vi "fake SampleRotator module.vi"(10 "Top":refnum<queue>, 11 "Rotator":refnum<queue>) -> (2 "deviceHandle":i32, 3 "Initialized":bool)   [LabVIEW 2022 SP3, in "SampleRotator.lvlib"]
doc: "This is a main VI of module for Sample rotator. It recives and executes commands, which comes from master controller. \nCommands and responses:\n\n/* */\nInitialize(path to driver DLL); -> Initialized(Contoller info<devN, devT, ID, Serial, Addr, connected?>);\n\n/* */\nUpdate(); -> Update(axis status<axis info, position, frequency, voltage>);\n\n/* */\nSetParameters(parameters<freq[Hz]; ampl[V]; offset[V]; tolerance[um]>); -> ParametersSet(parameters<freq; amp; offset; tolerance>);\n\n/* */\nSetPositon(positionToSet<relative?, double>) -> PositionSet(position to set<relative?, doubele);\n\n/* */\nEnd(), -> Disconnected();"
uses:
  SampleRotator.lvlib
  ctl/Rotator controller info.ctl
  ctl/Axis status.ctl
  Messenger service/Data types/Module name.ctl
  ctl/Motion Properties.ctl
  ctl/Positoin to set.ctl
  ctl/Rotator commands.ctl
panel:
  in  "Axis status in":T1={"Axis status"={"Connected"=TRUE, "Enabled"=FALSE, "Moving"=FALSE, "Target"=FALSE, "EndForward"=FALSE, "EndBackarwd"=FALSE, "Error"=FALSE}, "Position [°]"=0.0, "Frequency [Hz]"=1000.0, "Voltage [V]"=10.0, "Capacitance[uF]"=0.0, "Name"="", "ActuatorType"=0, "DC offset [V]"=0.0, "Tolerance [m°]"=0.0, "Index"=0} {"Index" items=["1", "2", "3"]; "ActuatorType" items=["Linear", "Rotator", "Goniometer"]}
  in  "controller info in":T2={"deviceNumber"=0, "DeviceType"=0, "ID"=0, "Serial"="", "Address"="FAKE", "connected"=TRUE} {"DeviceType" items=["ANC350res", "ANC350num", "ANC350fps", "No device / invalid"]; "ID" format="%x"}
  out "capacity":dbl
  out "wrong capacity":bool
  out "Axis status":T1 {"Index" items=["1", "2", "3"]; "ActuatorType" items=["Linear", "Rotator", "Goniometer"]}
  out "path to dll":path
  out "controller info":T2 {"DeviceType" items=["ANC350res", "ANC350num", "ANC350fps", "No device / invalid"]; "ID" format="%x"}
  out "ANC350v4 found":u32
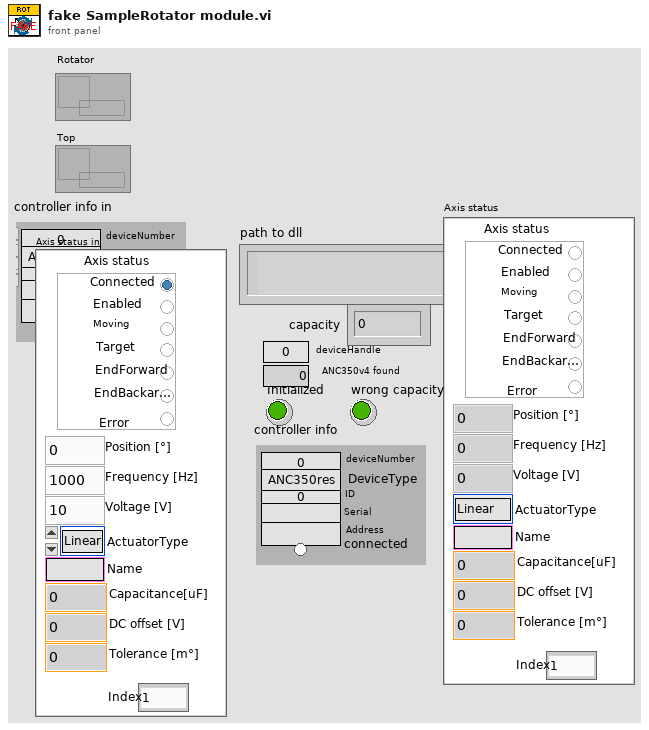
[diagram p1: front panel]
types:
  T1 = typedef "SampleRotator.lvlib/Axis status.ctl" = cluster{"Axis status":cluster{"Connected":bool, "Enabled":bool, "Moving":bool, "Target":bool, "EndForward":bool, "EndBackarwd":bool, "Error":bool}, "Position [°]":dbl, "Frequency [Hz]":dbl, "Voltage [V]":dbl, "Capacitance[uF]":dbl, "Name":string, "ActuatorType":u16, "DC offset [V]":dbl, "Tolerance [m°]":dbl, "Index":u8}
  T2 = typedef "SampleRotator.lvlib/Rotator controller info.ctl" = cluster{"deviceNumber":i32, "DeviceType":i32, "ID":u32, "Serial":string, "Address":string, "connected":bool}
  T3 = typedef "SampleRotator.lvlib/Rotator commands.ctl" = enum16{"Ignore", "Initialize", "Initialize axes", "Update", "Set parameters", "Stop movement", "Set position", "Disconnect", "End"}
  T4 = typedef "Module name.ctl" = enum16{"Emty", "Magnet", "VTI", "Excitation", "Servo", "Acquisition", "Rotator", "Digitizer", "SMU2450", "Carousel", "Multimeter", "Tmp monitor", "Power monitor"}
  T5 = typedef "Motion Properties.ctl" = cluster{"Frequency [Hz]":dbl, "MaxErr [µm|m°]":dbl, "DC voltage [V]":dbl, "Amplitude [V]":dbl, "Position [mm|°]":dbl, "EoF":bool, "EoB":bool, "Error":bool, "Target [mm|°]":dbl}
  T6 = typedef "Positoin to set.ctl" = cluster{"Relative?":bool, "Position [°]":dbl, "Safe to move?":bool}
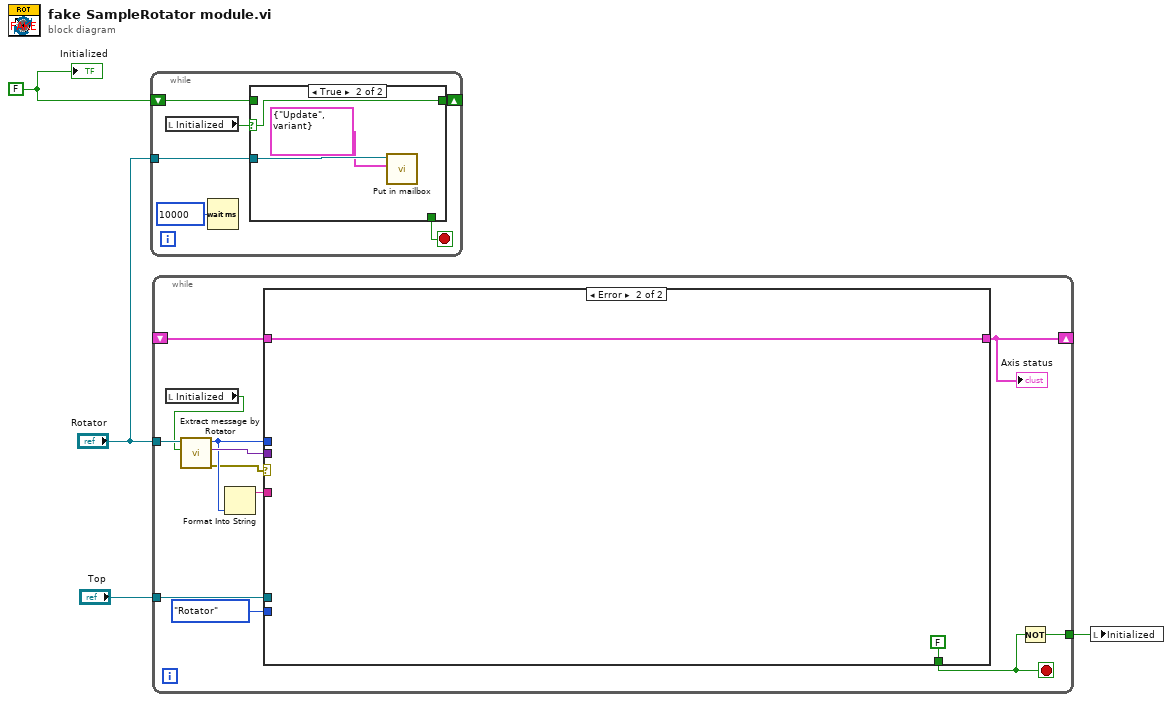
[diagram p0: block diagram]
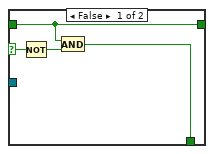
[diagram p2: hidden frame]
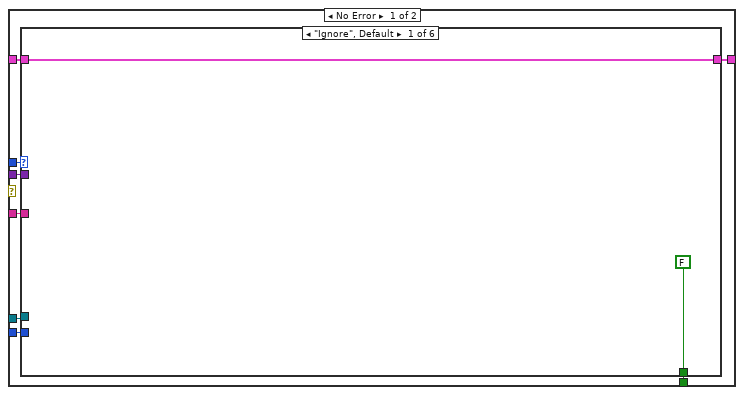
[diagram p3: hidden frame]
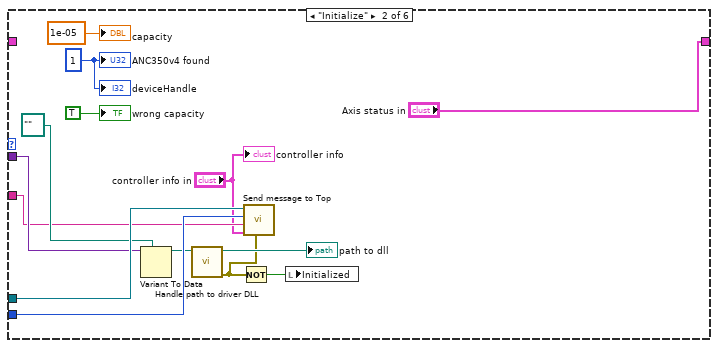
[diagram p4: hidden frame]
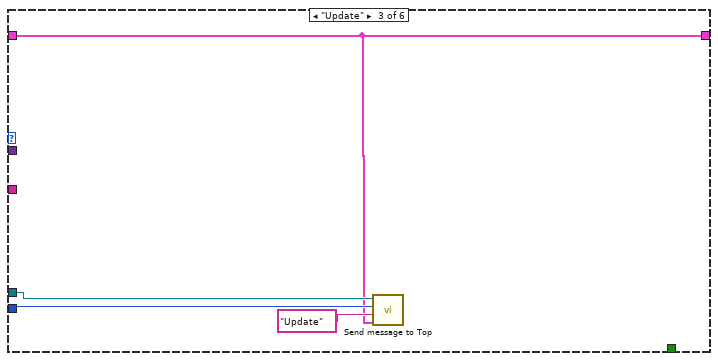
[diagram p5: hidden frame]
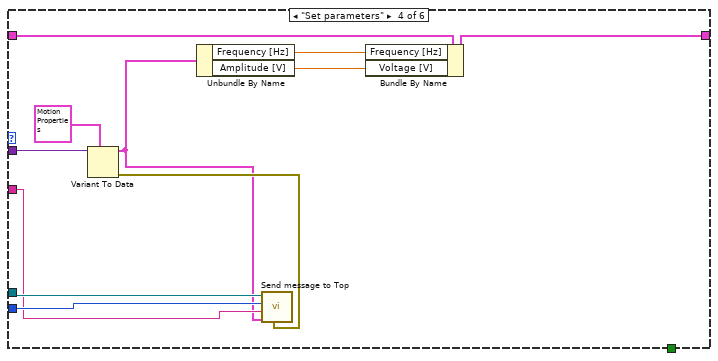
[diagram p6: hidden frame]
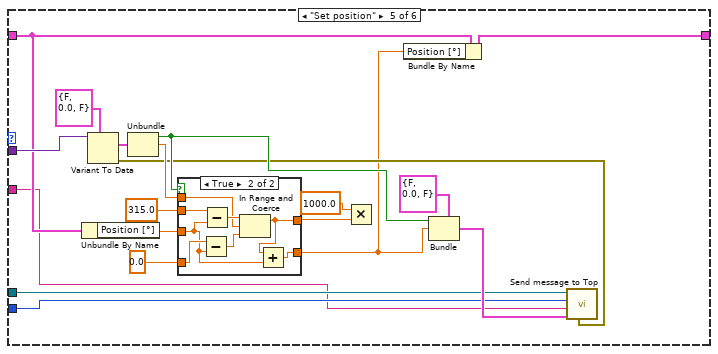
[diagram p7: hidden frame]
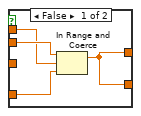
[diagram p8: hidden frame]
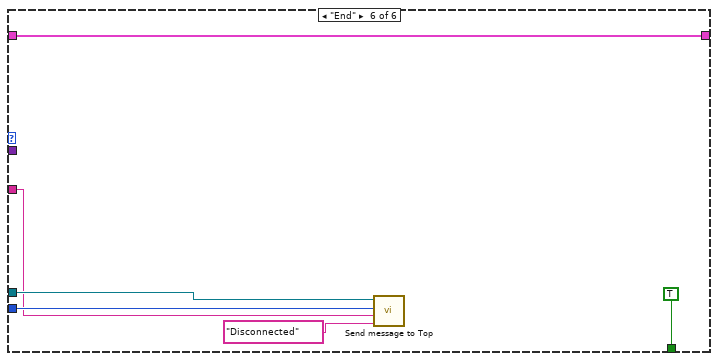
[diagram p9: hidden frame]
diagram:
  w4 = FALSE
  n1 = while {
    shift-right: [w8] -> _
    shift-left: w4 -> [w7]
    tunnel: "Rotator" -> [w5]
    stop <- w6 stop-if-true
    n2 = local read "Initialized"() -> (w10:bool)
    n3 = Wait (ms)(milliseconds to wait=u32 10000) -> ()  [unwired: 1 out]
    n4 = case shown="True" w10 {
      selector: w10 -> [w14 w17]
      tunnel: [w11 w17] -> w8
      tunnel: w7 -> [w11 _]
      tunnel: [w12 _] -> w6
      tunnel: w5 -> [_ w16]
      frame False {
        n5 = Not(x=w14) -> (.not. x?=w13:bool)
        n6 = And(x=w11, y=w13) -> (x .and. y?=w12:bool)
      }
      frame True {
        n7 = call "Put in mailbox.vi"("Message"=cluster{"Command":T3, "Data":variant} {"Command"=enum."Update", "Data"=variant} ("MSG to rotator"), "Queue in"=w16) -> ()  [unwired: 7 in, 3 out]
      }
    }
  }
  n8 = while {
    tunnel: "Rotator" -> [w27]
    tunnel: "Top" -> [w29]
    shift-right: [w25] -> _
    shift-left: _ -> [w24]
    tunnel: [w21] -> w1
    stop <- w22 stop-if-true
    n9 = local read "Initialized"() -> (w23:bool)
    n10 = call "Extract message by Rotator.vi"("Initialized?"=w23, "Queue in"=w27) -> ("error out"=w18:errorcluster, "Data"=w26:variant, "Command out"=w20:T3)  [unwired: 6 in, 1 out]
    n11 = Format Into String(w20) -> (resulting string=w19:string)  [unwired: 3 in, 1 out]
    n12 = case shown="Error" w18 {
      tunnel: w29 -> [w37 _]
      tunnel: Module_name."Rotator" ("Module name") -> [w36 _]
      tunnel: w26 -> [w35 _]
      tunnel: [w34 w107] -> w25
      tunnel: w24 -> [w33 w107]
      tunnel: [w32 FALSE] -> w22
      tunnel: w20 -> [w31 _]
      tunnel: w19 -> [w30 _]
      frame No Error {
        n13 = case shown="\"Ignore\", Default" w31 {
          tunnel: [FALSE _ _ _ _ TRUE] -> w32
          tunnel: w37 -> [_ w53 w57 w66 w75 w105]
          tunnel: w36 -> [_ w52 w56 w65 w76 w104]
          tunnel: w35 -> [_ w51 _ w67 w87 _]
          tunnel: [w38 "Axis status in" w54 w61 w70 w103] -> w34
          tunnel: w33 -> [w38 _ w54 w64 w85 w103]
          tunnel: w30 -> [_ w46 _ w63 w74 w100]
          frame "Ignore", Default {
          }
          frame "Initialize" {
            w40 = u32 1 ("ANC350v4 found")
            n14 = Variant To Data(type=path "", Variant=w51) -> (data=w49:path)  [unwired: 1 in, 1 out]
            n15 = call "Handle path to driver DLL.vi"("Path to DLL"=w49) -> ("error out"=w41:errorcluster, "path out"=→"path to dll":path)  [unwired: 9 in]
            n16 = Not(x=w41) -> (.not. x?=w47:bool)
            n17 = call "Send message to Top.vi"("Error in (no error)"=w41, "Data"="controller info in", "Response"=w46, "Module"=w52, "Mailbox address in"=w53) -> ()  [unwired: 5 in, 2 out]
            n18 = local write "Initialized"(w47) -> ()
            "ANC350v4 found" <- w40
            "controller info" <- "controller info in"
            "deviceHandle" <- w40
            "wrong capacity" <- TRUE ("wrong capacity")
            "capacity" <- 1e-05
          }
          frame "Update" {
            n19 = call "Send message to Top.vi"("Data"=w54, "Response"="Update", "Module"=w56, "Mailbox address in"=w57) -> ()  [unwired: 6 in, 2 out]
          }
          frame "Set parameters" {
            n20 = Variant To Data(type=T5 {"Frequency [Hz]"=1000.0, "MaxErr [µm|m°]"=10.0, "DC voltage [V]"=1.0, "Amplitude [V]"=6.0, "Position [mm|°]"=0.0, "EoF"=FALSE, "EoB"=FALSE, "Error"=FALSE, "Target [mm|°]"=0.0} ("Motion parameters"), Variant=w67) -> (data=w60:T5, error out=w62:errorcluster)  [unwired: 1 in]
            n21 = Unbundle By Name(w60) -> ("Frequency [Hz]"=w59:dbl, "Amplitude [V]"=w58:dbl)
            n22 = call "Send message to Top.vi"("Error in (no error)"=w62, "Data"=w60, "Response"=w63, "Module"=w65, "Mailbox address in"=w66) -> ()  [unwired: 5 in, 2 out]
            n23 = Bundle By Name(cluster=w64, "Frequency [Hz]"=w59, "Voltage [V]"=w58) -> (w61:T1)
          }
          frame "Set position" {
            n24 = Unbundle By Name(w85) -> ("Position [°]"=w83:dbl)
            n25 = Variant To Data(type=T6 {"Relative?"=FALSE, "Position [°]"=0.0, "Safe to move?"=FALSE}, Variant=w87) -> (data=w84:T6, error out=w71:errorcluster)  [unwired: 1 in]
            n26 = Unbundle(w84) -> ("Relative?"=w79:bool, "Position [°]"=w73:dbl)  [unwired: 1 out]
            n27 = case shown="True" w79 {
              tunnel: w73 -> [w89 w95]
              tunnel: w83 -> [_ w94]
              tunnel: [w88 w92] -> w78
              tunnel: 315.0 ("lower limit") -> [w91 w97]
              tunnel: 0.0 ("upper limit") -> [w90 w96]
              tunnel: [w88 w93] -> w69
              frame False {
                n28 = In Range and Coerce(upper limit=w91, x=w89, lower limit=w90) -> (coerced(x)=w88:dbl)  [unwired: 1 out]
              }
              frame True {
                n29 = Subtract(x=w96, y=w94) -> (x-y=w98:dbl)
                n30 = Subtract(x=w97, y=w94) -> (x-y=w99:dbl)
                n31 = In Range and Coerce(upper limit=w99, x=w95, lower limit=w98) -> (coerced(x)=w92:dbl)  [unwired: 1 out]
                n32 = Add(x=w92, y=w94) -> (x+y=w93:dbl)
              }
            }
            n33 = Multiply(x=1000.0, y=w78) -> ()  [unwired: 1 out]
            n34 = Bundle By Name(cluster=w85, "Position [°]"=w69) -> (w70:T1)
            n35 = Bundle(cluster=T6 {"Relative?"=FALSE, "Position [°]"=0.0, "Safe to move?"=FALSE}, "Relative?"=w79, "Position [°]"=w69) -> (w77:T6)  [unwired: 1 in]
            n36 = call "Send message to Top.vi"("Error in (no error)"=w71, "Data"=w77, "Response"=w74, "Module"=w76, "Mailbox address in"=w75) -> ()  [unwired: 5 in, 2 out]
          }
          frame "End" {
            n37 = call "Send message to Top.vi"("Data"="Disconnected" ("Response"), "Response"=w100, "Module"=w104, "Mailbox address in"=w105) -> ()  [unwired: 6 in, 2 out]
          }
        }
      }
      frame Error {
      }
    }
    "Axis status" <- w25
    n38 = Not(x=w22) -> (.not. x?=w21:bool)
  }
  n39 = local write "Initialized"(w1) -> ()
  "Initialized" <- w4
